vi "registerSaveEvent.vi"(8 "error in (no error)":errorcluster, 11 "ScriptEvent in":refnum<class "ScriptEvent.lvclass">) -> (0 "error out":errorcluster, 3 "ScriptEvent out":refnum<class "ScriptEvent.lvclass">)   [LabVIEW 2011, in "Events.lvlib" / "ScriptEvent.lvclass"]
uses:
  ScriptEvent.lvclass
  Event.lvclass
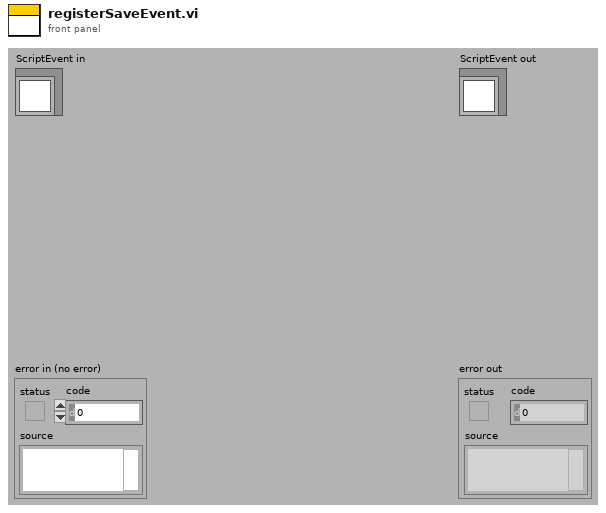
[diagram p1: front panel]
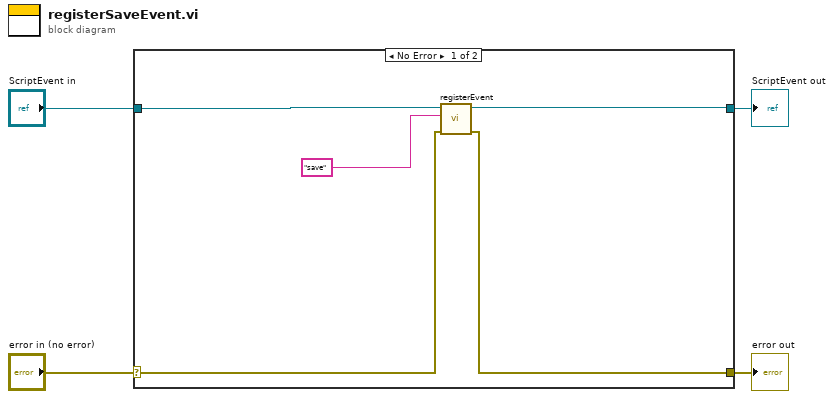
[diagram p0: block diagram]
diagram:
  n1 = case shown="No Error" "error in (no error)" {
    selector: "error in (no error)" -> [w7 w11]
    tunnel: [w6 w11] -> w3
    tunnel: [w5 w10] -> w1
    tunnel: "ScriptEvent in" -> [w9 w10]
    frame No Error {
      n2 = call "registerEvent.vi"("error in (no error)"=w7, "name"="save", "Event in"=w9) -> ("error out"=w6:errorcluster, "Event out"=w5:refnum<class "ScriptEvent.lvclass">)  [unwired: 7 in]
    }
    frame Error {
    }
  }
  "error out" <- w3
  "ScriptEvent out" <- w1
